vi "sv_Design Octave Filter Set.vi"(0 "scaled signal [EU]":waveform(dbl), 5 "1/n octave settings":T4, 7 "band number":cluster{"low band":i32, "high band":i32}, 11 "error in (no error)":errorcluster) -> (4 "dup scaled signal [EU]":waveform(dbl), 6 "filter bank parameters":T2={"octave filter coefficients"=[{"filter structure"=enum."IIR 2nd Order", "Reverse Coefficients"=[1.0], "Forward Coefficients"=[]}], "lowpass filter coefficients"={"filter structure"=enum."IIR 2nd Order", "Reverse Coefficients"=[], "Forward Coefficients"=[]}, "number of samples to settle"=0, "number of decimation steps required"=[], "octave filter bandwidth"=[]}, 8 "initialize filter state":T1, 10 "nominal frequencies [Hz]":dbl[](array[numeric]) format="%.2f", 15 "error out":errorcluster)   [LabVIEW 2017, in "SoundVib_Octave_2014 standard.lvlib"]
uses:
  <vilib>/addons/Sound and Vibration/svt_Octave/SoundVib_Octave_2014 standard.lvlib
  <vilib>/addons/_NISVFA/_Shared subVIs/Controls/svc_Octave Standard.ctl
  <vilib>/addons/_NISVFA/_Shared subVIs/Controls/svc_Octave Filter Bank Parameters.ctl
  <vilib>/addons/_NISVFA/_Shared subVIs/Controls/svc_Octave Filter State.ctl
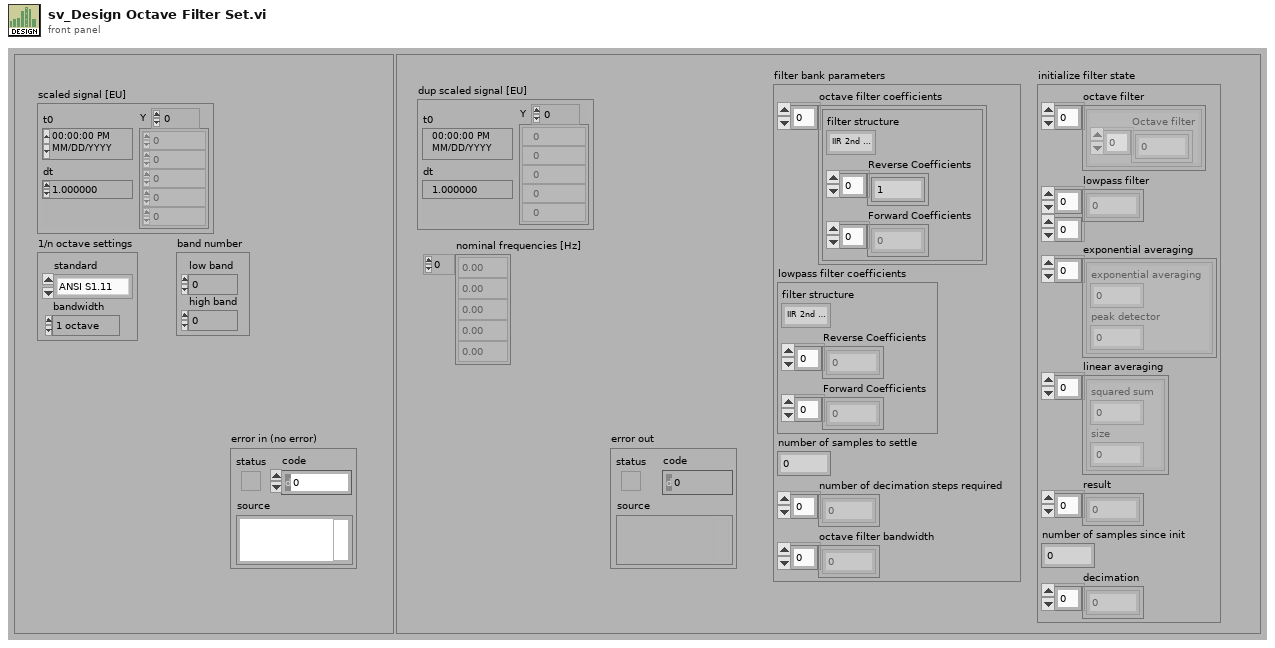
[diagram p1: front panel]
types:
  T1 = typedef "svc_Octave Filter State.ctl" = cluster{"octave filter":cluster{"Octave filter":dbl[]}[], "lowpass filter":dbl[][], "exponential averaging":cluster{"exponential averaging":dbl, "peak detector":dbl}[], "linear averaging":cluster{"squared sum":dbl, "size":dbl}[], "result":dbl[], "number of samples since init":u64, "decimation":dbl[]}
  T2 = typedef "svc_Octave Filter Bank Parameters.ctl" = cluster{"octave filter coefficients":cluster{"filter structure":enum32{"IIR 2nd Order", "IIR 4th Order"}, "Reverse Coefficients":dbl[], "Forward Coefficients":dbl[]}[], "lowpass filter coefficients":cluster{"filter structure":enum32{"IIR 2nd Order", "IIR 4th Order"}, "Reverse Coefficients":dbl[], "Forward Coefficients":dbl[]}, "number of samples to settle":u64, "number of decimation steps required":i32[], "octave filter bandwidth":dbl[]}
  T3 = typedef "svc_Octave Standard.ctl" = enum16{"ANSI S1.11", "IEC 61260"}
  T4 = cluster{"standard":T3, "bandwidth":enum16{"1 octave", "1/3 octave", "1/6 octave", "1/12 octave", "1/24 octave"}}
  T5 = enum16{"1 octave", "1/3 octave", "1/6 octave", "1/12 octave", "1/24 octave"}
  T6 = cluster{"octave filter":cluster{"Octave filter":dbl[]}[], "decimation":i32[], "lowpass filter":dbl[][], "exponential averaging":cluster{"exponential averaging":dbl, "peak detector":dbl}[], "linear averaging":cluster{"squared sum":dbl, "size":dbl}[], "result":dbl[], "# samples since init":u64}
  T7 = cluster{"# special filters":i32, "special filter coefficients":cluster{"filter structure":enum32{"IIR 2nd Order", "IIR 4th Order"}, "Reverse Coefficients":dbl[], "Forward Coefficients":dbl[]}[], "# filters per octave":cluster{"# filters":i32, "starting at":i32}[], "standard filter coefficients":cluster{"filter structure":enum32{"IIR 2nd Order", "IIR 4th Order"}, "Reverse Coefficients":dbl[], "Forward Coefficients":dbl[]}[], "# decimation steps":i32, "lowpass filter coefficients":cluster{"filter structure":enum32{"IIR 2nd Order", "IIR 4th Order"}, "Reverse Coefficients":dbl[], "Forward Coefficients":dbl[]}, "# samples to settle":u64, "special filter bandwidth":dbl[], "standard filter bandwidth":dbl[]}
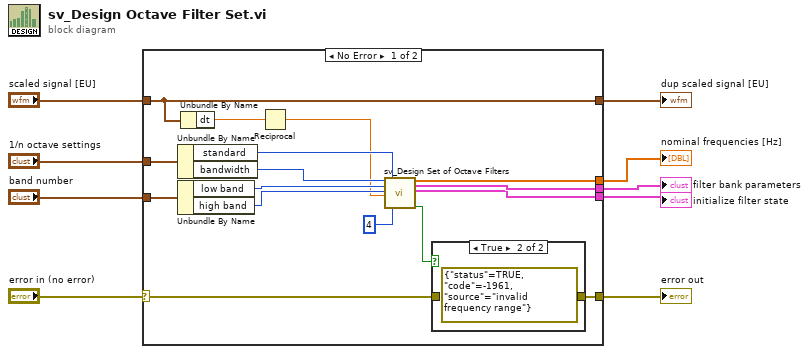
[diagram p0: block diagram]
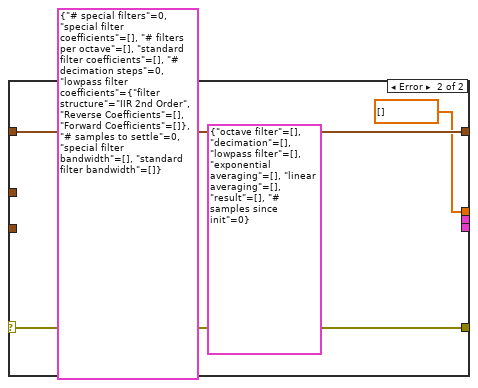
[diagram p3: hidden frame]
diagram:
  n1 = case shown="No Error" "error in (no error)" {
    selector: "error in (no error)" -> [w16 w28]
    tunnel: [w25 dbl[] [] ("nominal frequencies [Hz]")] -> w9
    tunnel: "band number" -> [w24 _]
    tunnel: "1/n octave settings" -> [w23 _]
    tunnel: "scaled signal [EU]" -> [w18 w30]
    tunnel: [w17 w28] -> w4
    tunnel: [w18 w30] -> w3
    tunnel: [w12 _] -> w2
    tunnel: [w11 _] -> w1
    frame No Error {
      n2 = Unbundle By Name(w23) -> ("standard"=w14:T3, "bandwidth"=w19:T5)
      n3 = Unbundle By Name(w24) -> ("low band"=w20:i32, "high band"=w21:i32)
      n4 = Unbundle By Name(w18) -> ("dt"=w22:dbl)
      n5 = Reciprocal(x=w22) -> (1/x=w13:dbl)
      n6 = call <vilib>:"sv_Design Set of Octave Filters.vi"("bandwidth"=w19, "low band selector"=w20, "high band selector"=w21, "sampling frequency [Hz]"=w13, "standard"=w14, "Butterworth filter order"=4) -> ("nominal frequencies [Hz]"=w25:dbl[], "filter bank parameters"=w12:T2, "initialize filter state"=w11:T1, "error"=w15:bool)  [unwired: 8 in, 2 out]
      n7 = case shown="True" w15 {
        tunnel: w16 -> [w26 _]
        tunnel: [w26 errorcluster {"status"=TRUE, "code"=-1961, "source"="invalid frequency range"} ("error IO")] -> w17
        frame False {
        }
        frame True {
        }
      }
    }
    frame Error {
      (unwired) T6 {"octave filter"=[], "decimation"=[], "lowpass filter"=[], "exponential averaging"=[], "linear averaging"=[], "result"=[], "# samples since init"=0} ("initialize filter state")
      (unwired) T7 {"# special filters"=0, "special filter coefficients"=[], "# filters per octave"=[], "standard filter coefficients"=[], "# decimation steps"=0, "lowpass filter coefficients"={"filter structure"=enum."IIR 2nd Order", "Reverse Coefficients"=[], "Forward Coefficients"=[]}, "# samples to settle"=0, "special filter bandwidth"=[], "standard filter bandwidth"=[]} ("filter bank parameters")
    }
  }
  "nominal frequencies [Hz]" <- w9
  "error out" <- w4
  "dup scaled signal [EU]" <- w3
  "filter bank parameters" <- w2
  "initialize filter state" <- w1
